vi "NanoOps.vi"(8 "error in (no error)":errorcluster, 9 "Serial open (T)?":bool=TRUE, 10 "Toggle time Msecs":dbl, 11 "Cmd":T1) -> (0 "error out":errorcluster={"status"=FALSE, "code"=1073676294, "source"="VISA Read in DoNanoCmd.vi"}, 2 "Return data":dbl, 3 "Nano out":refnum<visa-resource-name>="COM20")   [LabVIEW 2013]
uses:
  Nano_commands.ctl
  NanoCmds.ctl
  Test Globals/Global 1.vi
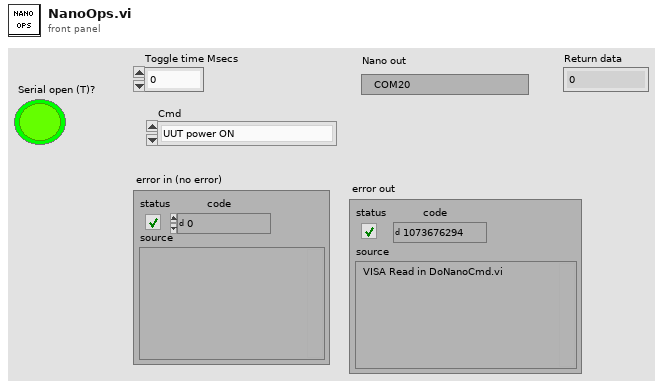
[diagram p1: front panel]
types:
  T1 = typedef "Nano_commands.ctl" = enum16{"UUT power ON", "UUT power OFF", "Get current draw", "Toggle ON_OFF", "Toggle nReset", "ADC .832vdc", "ADC 0vdc", "Read CTS", "Read nSleep", "Init", "Wait for lid to be closed", "Power up, start, get current", "Wait for lid open", "Check if X2 shorted", "Power up and start up", "Check X3 shorted"}
  T2 = typedef "NanoCmds.ctl" = enum16{"Make digital port an output", "Make digital port an input", "Set digital pin high", "Set digital pin low", "Get digital pin state", "Get analog pin voltage", "Get analog pins difference", "Get ohms at analog pin", "Turn on current limit", "Reset Nano device", "Get digital pin state pullup", "Read current", "Initialize", "Power up uut", "Power down uut", "Get uut current draw", "Set ADC volts high", "Set ADC volts low", "Start up uut modem", "Get CTS state", "Get on_nsleep state", "Reset modem", "Get lid state", "Wait for lid closed", "Wait for lid open", "Power up, start, get curr", "Check if X2 shorted", "Power up and start up", "Check X3 shorted", "Get RTS state", "Get DTR state", "Reboot 1002759"}
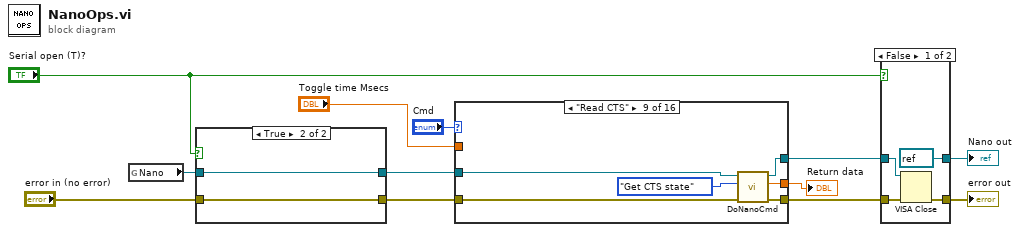
[diagram p0: block diagram]
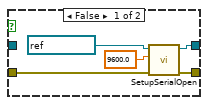
[diagram p3: hidden frame]
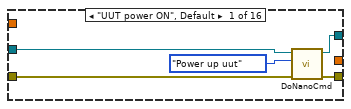
[diagram p4: hidden frame]
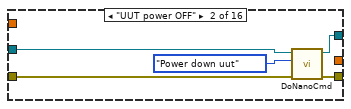
[diagram p5: hidden frame]
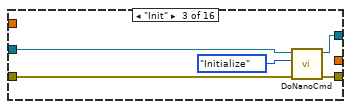
[diagram p6: hidden frame]
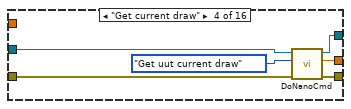
[diagram p7: hidden frame]
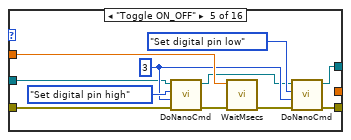
[diagram p8: hidden frame]
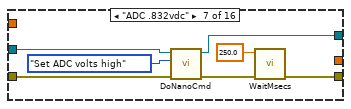
[diagram p10: hidden frame]
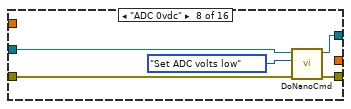
[diagram p11: hidden frame]
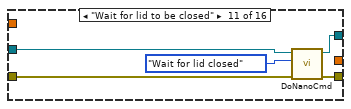
[diagram p13: hidden frame]
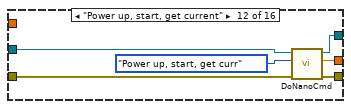
[diagram p14: hidden frame]
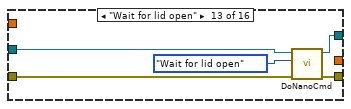
[diagram p15: hidden frame]
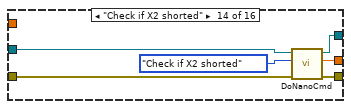
[diagram p16: hidden frame]
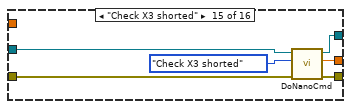
[diagram p17: hidden frame]
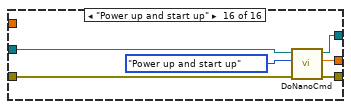
[diagram p18: hidden frame]
diagram:
  n1 = global read "Global 1.vi" "Nano"() -> (w8:refnum<visa-resource-name>)
  n2 = case shown="True" "Serial open (T)?" {
    tunnel: "error in (no error)" -> [w17 w18]
    tunnel: [w14 w19] -> w7
    tunnel: [w13 w18] -> w2
    tunnel: w8 -> [_ w19]
    frame False {
      n3 = call "SetupSerialOpen.vi"("error in (no error)"=w17, "Baud"=9600.0, "VISA Refnum in"=refnum<visa-resource-name> "COM21") -> ("error out"=w13:errorcluster, "VISA session"=w14:refnum<visa-resource-name>)  [unwired: 7 in]
    }
    frame True {
    }
  }
  n4 = case shown="\"Read CTS\"" "Cmd" {
    tunnel: [w23 w29 w34 w40 w50 w53 w57 w64 w71 w73 w78 w84 w89 w94 w100 w107] -> w6
    tunnel: "Toggle time Msecs" -> [_ _ _ _ w46 _ _ _ _ _ _ _ _ _ _ _]
    tunnel: [w22 w27 w32 w39 w49 w52 w59 w63 w70 w72 w77 w83 w88 w93 w99 w106] -> w4
    tunnel: [_ _ _ w37 _ _ _ _ w68 _ _ w82 _ w92 w98 w105] -> w10
    tunnel: w7 -> [w20 w25 w30 w35 w41 w52 w55 w61 w66 w72 w74 w79 w85 w90 w96 w102]
    tunnel: w2 -> [w21 w26 w31 w36 w42 w53 w54 w62 w67 w73 w75 w80 w86 w91 w97 w103]
    frame "UUT power ON", Default {
      n5 = call "DoNanoCmd.vi"("error in (no error)"=w21, "Nano Op"=NanoCmds."Power up uut", "VISA resource name"=w20) -> ("error out"=w23:errorcluster, "VISA resource name 2"=w22:refnum<visa-resource-name>)  [unwired: 5 in, 2 out]
    }
    frame "UUT power OFF" {
      n6 = call "DoNanoCmd.vi"("error in (no error)"=w26, "Nano Op"=NanoCmds."Power down uut", "VISA resource name"=w25) -> ("error out"=w29:errorcluster, "VISA resource name 2"=w27:refnum<visa-resource-name>)  [unwired: 5 in, 2 out]
    }
    frame "Init" {
      n7 = call "DoNanoCmd.vi"("error in (no error)"=w31, "Nano Op"=NanoCmds."Initialize", "VISA resource name"=w30) -> ("error out"=w34:errorcluster, "VISA resource name 2"=w32:refnum<visa-resource-name>)  [unwired: 5 in, 2 out]
    }
    frame "Get current draw" {
      n8 = call "DoNanoCmd.vi"("error in (no error)"=w36, "Nano Op"=NanoCmds."Get uut current draw", "VISA resource name"=w35) -> ("error out"=w40:errorcluster, "Read Value"=w37:dbl, "VISA resource name 2"=w39:refnum<visa-resource-name>)  [unwired: 5 in, 1 out]
    }
    frame "Toggle ON_OFF" {
      w44 = u32 3 ("Pin 1")
      n9 = call "DoNanoCmd.vi"("error in (no error)"=w42, "Pin 1"=w44, "Nano Op"=NanoCmds."Set digital pin high", "VISA resource name"=w41) -> ("error out"=w47:errorcluster, "VISA resource name 2"=w43:refnum<visa-resource-name>)  [unwired: 4 in, 2 out]
      n10 = call "WaitMsecs.vi"("error in (no error)"=w47, "Wait Msecs"=w46) -> ("error out"=w45:errorcluster)  [unwired: 9 in]
      n11 = call "DoNanoCmd.vi"("error in (no error)"=w45, "Pin 1"=w44, "Nano Op"=NanoCmds."Set digital pin low", "VISA resource name"=w43) -> ("error out"=w50:errorcluster, "VISA resource name 2"=w49:refnum<visa-resource-name>)  [unwired: 4 in, 2 out]
    }
    frame "Toggle nReset" {
    }
    frame "ADC .832vdc" {
      n12 = call "DoNanoCmd.vi"("error in (no error)"=w54, "Nano Op"=NanoCmds."Set ADC volts high", "VISA resource name"=w55) -> ("error out"=w58:errorcluster, "VISA resource name 2"=w59:refnum<visa-resource-name>)  [unwired: 5 in, 2 out]
      n13 = call "WaitMsecs.vi"("error in (no error)"=w58, "Wait Msecs"=250.0) -> ("error out"=w57:errorcluster)  [unwired: 9 in]
    }
    frame "ADC 0vdc" {
      n14 = call "DoNanoCmd.vi"("error in (no error)"=w62, "Nano Op"=NanoCmds."Set ADC volts low", "VISA resource name"=w61) -> ("error out"=w64:errorcluster, "VISA resource name 2"=w63:refnum<visa-resource-name>)  [unwired: 5 in, 2 out]
    }
    frame "Read CTS" {
      n15 = call "DoNanoCmd.vi"("error in (no error)"=w67, "Nano Op"=NanoCmds."Get CTS state", "VISA resource name"=w66) -> ("error out"=w71:errorcluster, "Read Value"=w68:dbl, "VISA resource name 2"=w70:refnum<visa-resource-name>)  [unwired: 5 in, 1 out]
    }
    frame "Read nSleep" {
    }
    frame "Wait for lid to be closed" {
      n16 = call "DoNanoCmd.vi"("error in (no error)"=w75, "Nano Op"=NanoCmds."Wait for lid closed", "VISA resource name"=w74) -> ("error out"=w78:errorcluster, "VISA resource name 2"=w77:refnum<visa-resource-name>)  [unwired: 5 in, 2 out]
    }
    frame "Power up, start, get current" {
      n17 = call "DoNanoCmd.vi"("error in (no error)"=w80, "Nano Op"=NanoCmds."Power up, start, get curr", "VISA resource name"=w79) -> ("error out"=w84:errorcluster, "Read Value"=w82:dbl, "VISA resource name 2"=w83:refnum<visa-resource-name>)  [unwired: 5 in, 1 out]
    }
    frame "Wait for lid open" {
      n18 = call "DoNanoCmd.vi"("error in (no error)"=w86, "Nano Op"=NanoCmds."Wait for lid open", "VISA resource name"=w85) -> ("error out"=w89:errorcluster, "VISA resource name 2"=w88:refnum<visa-resource-name>)  [unwired: 5 in, 2 out]
    }
    frame "Check if X2 shorted" {
      n19 = call "DoNanoCmd.vi"("error in (no error)"=w91, "Nano Op"=NanoCmds."Check if X2 shorted", "VISA resource name"=w90) -> ("error out"=w94:errorcluster, "Read Value"=w92:dbl, "VISA resource name 2"=w93:refnum<visa-resource-name>)  [unwired: 5 in, 1 out]
    }
    frame "Check X3 shorted" {
      n20 = call "DoNanoCmd.vi"("error in (no error)"=w97, "Nano Op"=NanoCmds."Check X3 shorted", "VISA resource name"=w96) -> ("error out"=w100:errorcluster, "Read Value"=w98:dbl, "VISA resource name 2"=w99:refnum<visa-resource-name>)  [unwired: 5 in, 1 out]
    }
    frame "Power up and start up" {
      n21 = call "DoNanoCmd.vi"("error in (no error)"=w103, "Nano Op"=NanoCmds."Power up and start up", "VISA resource name"=w102) -> ("error out"=w107:errorcluster, "Read Value"=w105:dbl, "VISA resource name 2"=w106:refnum<visa-resource-name>)  [unwired: 5 in, 1 out]
    }
  }
  "Return data" <- w10
  n22 = case shown="False" "Serial open (T)?" {
    tunnel: w6 -> [w111 w113]
    tunnel: [w110 w113] -> w5
    tunnel: w4 -> [w109 w112]
    tunnel: [refnum<visa-resource-name> refnum ("VISA resource name 2") w112] -> w3
    frame False {
      n23 = VISA Close(VISA resource name=w109, error in (no error)=w111) -> (error out=w110:errorcluster)
    }
    frame True {
    }
  }
  "error out" <- w5
  "Nano out" <- w3
